vi "Set Engine Offset.vi"(10 "engine offset":u64, 11 "Framework in":refnum<class "Framework.lvclass">) -> (3 "Framework out":refnum<class "Framework.lvclass">)   [LabVIEW 2019, in "DSF Core.lvlib" / "Framework.lvclass"]
uses:
  Framework.lvclass
  Framework.lvclass/Framework.ctl
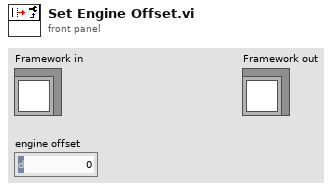
[diagram p1: front panel]
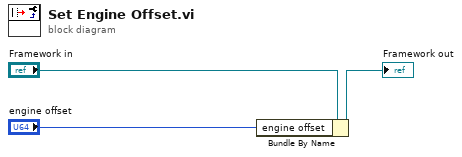
[diagram p0: block diagram]
diagram:
  n1 = Bundle By Name(cluster="Framework in", "engine offset"="engine offset") -> (→"Framework out":refnum<class "Framework.lvclass">)
